vi "1.4.vi"() -> ()   [LabVIEW 2013]
panel:
  out "Temperatura Convertida":dbl
  in  "Temperatura a Convertir":dbl
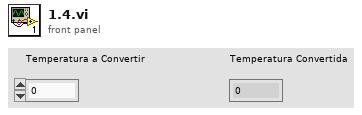
[diagram p1: front panel]
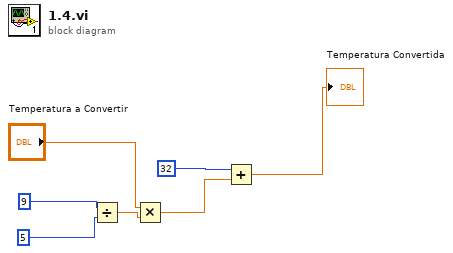
[diagram p0: block diagram]
diagram:
  n1 = Divide(x=9, y=5) -> (x/y=w3:dbl)
  n2 = Multiply(x="Temperatura a Convertir", y=w3) -> (x*y=w4:dbl)
  n3 = Add(x=32, y=w4) -> (x+y=→"Temperatura Convertida":dbl)
